vi "Get Vector.vi"(6 "no transpose\nfor reading":bool, 8 "error in (no error)":errorcluster, 9 "octave vector sizes":i32[](array[numeric]), 10 "variable name":string, 11 "pipe in":T1) -> (0 "error out":errorcluster, 2 "vector":string[](array[string]), 3 "pipe out":T1)   [LabVIEW 2013, in "GOLPI library.lvlib"]
doc: "Reads vector variable containing doubles from GNU Octave."
uses:
  GOLPI library.lvlib
  LV Process.lvlibp/Pipe Handle.ctl
  Globals.vi
  <vilib>/Utility/error.llb/Error Cluster From Error Code.vi
  <vilib>/ErrorRing/Error Ring.xnode
  LV Process.lvlibp
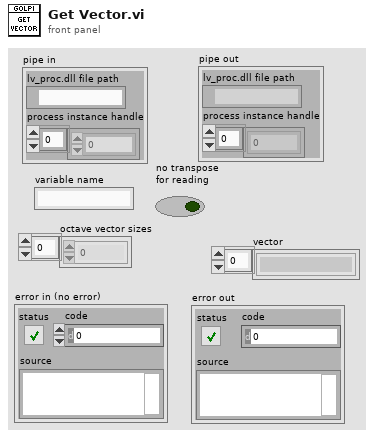
[diagram p1: front panel]
types:
  T1 = typedef "LV Process.lvlibp/Pipe Handle.ctl" = cluster{"lv_proc.dll file path":path, "process instance handle":u32[]}
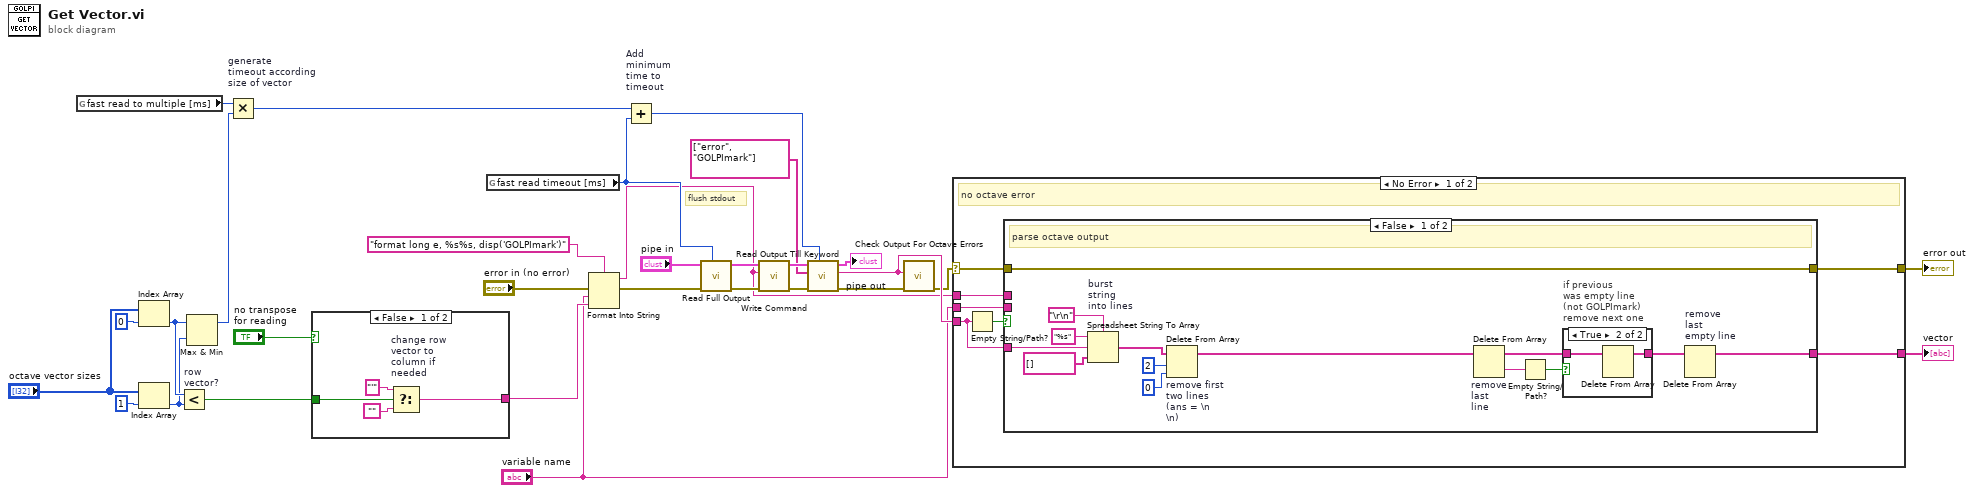
[diagram p0: block diagram]
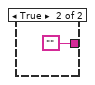
[diagram p2: hidden frame]
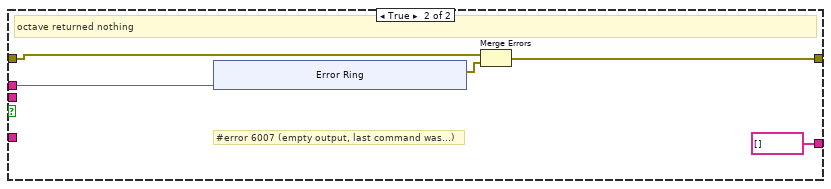
[diagram p4: hidden frame]
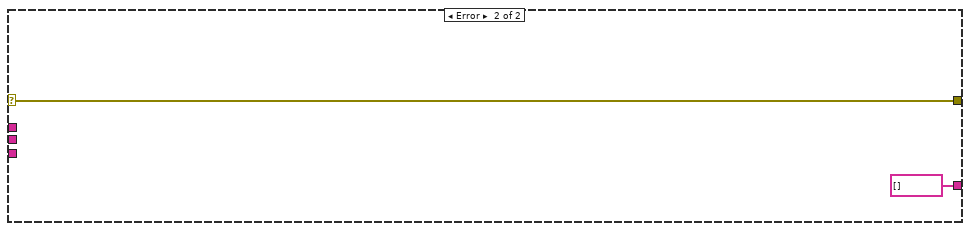
[diagram p5: hidden frame]
diagram:
  # "flush stdout"
  n1 = global read "Globals.vi" "fast read to multiple [ms]"() -> (w9:u32)
  n2 = Index Array(array="octave vector sizes", index=0) -> (element=w24:i32)
  n3 = Index Array(array="octave vector sizes", index=1) -> (element=w23:i32)
  n4 = Less? "row\nvector?"(x=w24, y=w23) -> (x < y?=w2:bool)
  n5 = Max & Min(x=w24, y=w23) -> (max(x,y)=w22:i32)  [unwired: 1 out]
  n6 = Multiply "generate\ntimeout according\nsize of vector"(x=w9, y=w22) -> (x*y=w16:u32)
  n7 = case shown="False" "no transpose\nfor reading" {
    tunnel: [w32 ""] -> w20
    tunnel: w2 -> [w31 _]
    frame False {
      n8 = Select "change row\nvector to\ncolumn if\nneeded"(t="'", s=w31, f="") -> (s? t:f=w32:string)
    }
    frame True {
    }
  }
  n9 = global read "Globals.vi" "fast read timeout [ms]"() -> (w10:u32)
  n10 = Format Into String(format string="format long e, %s%s, disp('GOLPImark')", error in="error in (no error)", "variable name", w20) -> (resulting string=w3:string, error out=w11:errorcluster)  [unwired: 1 in]
  n11 = Add "Add\nminimum\ntime to\ntimeout"(x=w16, y=w10) -> (x+y=w15:u32)
  n12 = call "Read Full Output.vi"("timeout [ms]"=w10, "error in"=w11, "pipe in"="pipe in") -> ("error out"=w12:errorcluster, "pipe out"=w13:T1)  [unwired: 5 in, 2 out]
  n13 = call "Write Command.vi"("error in"=w12, "command"=w3, "pipe in"=w13) -> ("error out"=w17:errorcluster, "pipe out"=w28:T1)  [unwired: 7 in]
  n14 = call "Read Output Till Keyword.vi"("timeout [ms]"=w15, "error in"=w17, "keywords"=string[] ["error", "GOLPImark"], "pipe in"=w28) -> ("error out"=w30:errorcluster, "read buffer"=w8:string, "pipe out"=→"pipe out":T1)  [unwired: 4 in, 1 out]
  n15 = call "Check Output For Octave Errors.vi"("error in"=w30, "read buffer"=w8) -> ("error out"=w4:errorcluster)  [unwired: 9 in]
  n16 = case shown="No Error" w4 {
    selector: w4 -> [w39 w73]
    tunnel: w8 -> [w38 _]
    tunnel: "variable name" -> [w42 _]
    tunnel: [w41 string[] []] -> w6
    tunnel: [w40 w73] -> w5
    tunnel: w3 -> [w36 _]
    frame No Error {
      # "no octave error"
      n17 = Empty String/Path?(string/path=w38) -> (empty?=w37:bool)
      n18 = case shown="False" w37 {
        tunnel: w38 -> [w52 _]
        tunnel: w42 -> [_ _]
        tunnel: [w43 string[] []] -> w41
        tunnel: w39 -> [w56 w64]
        tunnel: [w56 w62] -> w40
        tunnel: w36 -> [_ w61]
        frame False {
          # "parse octave output"
          n19 = Spreadsheet String To Array "burst\nstring\ninto lines"(delimiter (Tab)="\r\n", format string="%s", spreadsheet string=w52, array type (2D Dbl)=string[] []) -> (array=w51:string[])
          n20 = Delete From Array "remove first\ntwo lines\n(ans = \\n\n\\n)"(array=w51, length=2, index=0) -> (array with subset deleted=w48:string[])  [unwired: 1 out]
          n21 = Delete From Array "remove\nlast\nline"(array=w48) -> (deleted portion=w47:string, array with subset deleted=w46:string[])  [unwired: 2 in]
          n22 = Empty String/Path?(string/path=w47) -> (empty?=w44:bool)
          n23 = case "if previous\nwas empty line\n(not GOLPImark)\nremove next one" shown="True" w44 {
            tunnel: w46 -> [w57 w59]
            tunnel: [w57 w58] -> w45
            frame False {
            }
            frame True {
              n24 = Delete From Array(array=w59) -> (array with subset deleted=w58:string[])  [unwired: 2 in, 1 out]
            }
          }
          n25 = Delete From Array "remove\nlast\nempty line"(array=w45) -> (array with subset deleted=w43:string[])  [unwired: 2 in, 1 out]
        }
        frame True {
          # "#error 6007 (empty output, last command was...)"
          # "octave returned nothing"
          n26 = xnode "Error Ring"("parameter 0"=w61) -> ("error out"=w63:errorcluster)
          n27 = Merge Errors(w64, w63) -> (w62:errorcluster)
        }
      }
    }
    frame Error {
    }
  }
  "error out" <- w5
  "vector" <- w6
